vi "readexcel.vi"() -> ()   [LabVIEW 2015]
uses:
  <vilib>/Utility/file.llb/Read Delimited Spreadsheet (DBL).vi
panel:
  out "mean2":dbl[][](array[numeric])
  out "mean1":dbl[][](array[numeric])
  out "array w/ subset deleted":dbl[][](array[numeric])
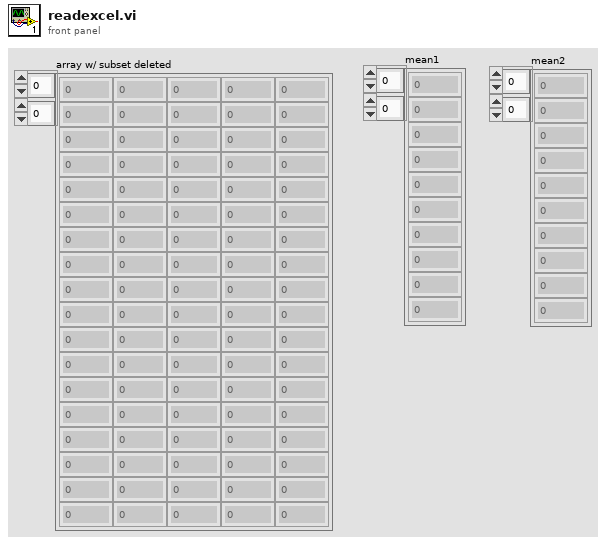
[diagram p1: front panel]
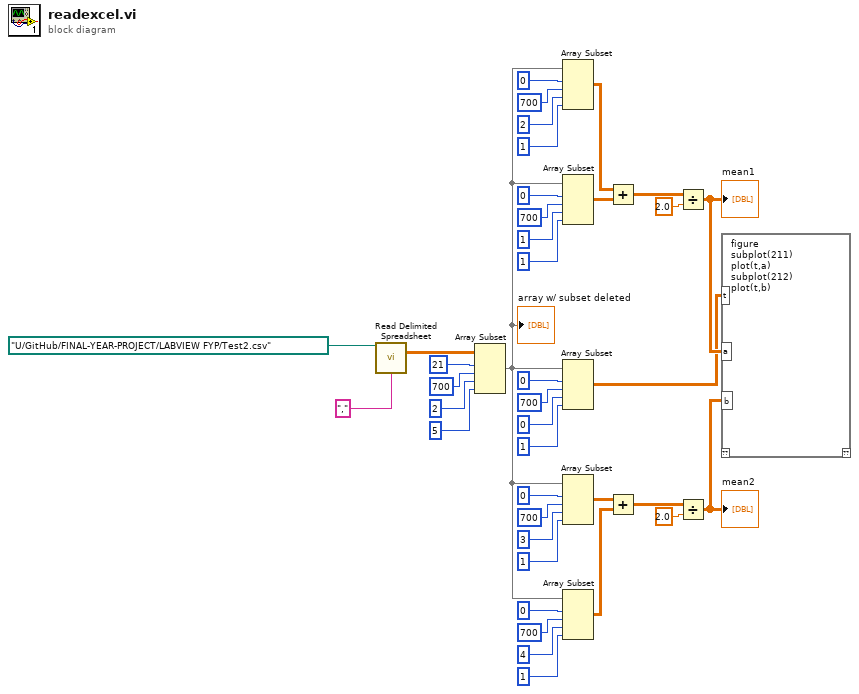
[diagram p0: block diagram]
diagram:
  n1 = call-poly <vilib>:"Read Delimited Spreadsheet.vi"("file path (dialog if empty)"=path "U:/GitHub/FINAL-YEAR-PROJECT/LABVIEW FYP/Test2.csv", "delimiter (\\t)"="," ("delimiter (\\t)")) -> ("all rows"=w37:dbl[][])  [unwired: 8 in, 5 out]
  n2 = Array Subset(array=w37, index (row)=21 ("index"), length (row)=700 ("index"), index (col)=2 ("index"), length (col)=5 ("index")) -> (w2:dbl[][])
  "array w/ subset deleted" <- w2
  n3 = Array Subset(array=w2, index (row)=0 ("index"), length (row)=700 ("length"), index (col)=2 ("index"), length (col)=1 ("length")) -> (w24:dbl[][])
  n4 = Array Subset(array=w2, index (row)=0 ("index"), length (row)=700 ("length"), index (col)=1 ("index"), length (col)=1 ("length")) -> (w23:dbl[][])
  n5 = Array Subset(array=w2, index (row)=0 ("index"), length (row)=700 ("length"), index (col)=0 ("index"), length (col)=1 ("length")) -> (w1:dbl[][])
  n6 = Array Subset(array=w2, index (row)=0 ("index"), length (row)=700 ("length"), index (col)=3 ("index"), length (col)=1 ("length")) -> (w21:dbl[][])
  n7 = Array Subset(array=w2, index (row)=0 ("index"), length (row)=700 ("length"), index (col)=4 ("index"), length (col)=1 ("length")) -> (w22:dbl[][])
  n8 = Add(x=w24, y=w23) -> (x+y=w9:dbl[][])
  n9 = Add(x=w21, y=w22) -> (x+y=w10:dbl[][])
  n10 = Divide(x=w9, y=2.0) -> (x/y=w8:dbl[][])
  "mean1" <- w8
  n11 = Divide(x=w10, y=2.0) -> (x/y=w7:dbl[][])
  "mean2" <- w7
  n12 = script code="figure\nsubplot(211)\nplot(t,a)\nsubplot(212)\nplot(t,b)"("a"=w8, "b"=w7, "t"=w1) -> ()  [unwired: 1 in, 1 out]
